vi "SUB_Get GUID.vi"() -> (0 "GUID OLE String":string, 1 "GUID String":string, 3 "GUID Cluster":T1 {"Data4" format="%.0x"; "Data3" format="%.0x"; "Data2" format="%.0x"; "Data1" format="%.0x"})   [LabVIEW 2015]
doc: "GUID stands for <B>G</B>lobally <B>U</B>nique <B>ID</B>entifier, a 128-bit integer used as unique identifier.\n\nThis VI makes a call to ole32.dll to create an absolutely unique number that you can use as a persistent identifier in a distributed environment.To a very high degree of certainty, this function returns a unique value: no other invocation, on the same or any other system (networked or not), should return the same value.\n\n<B>GUID Cluster</B> returns the GUID in a cluster that follows the GUID format.\n\n<B>GUID String</B> has the GUID as a string of characters.\n\n<B>GUID OLE String</B> has a format like that of the following sample:\n\n{c200e360-38c5-11ce-ae62-08002b2b79ef} \n \nwhere the successive fields break the GUID into the form:\n\nDWORD-WORD-WORD-WORD-WORD-DWORD\n\ncovering the 128-bit GUID. The string includes the enclosing braces, which are an OLE convention.\n\nEnrique Vargas\nvargas@jyestudio.com"
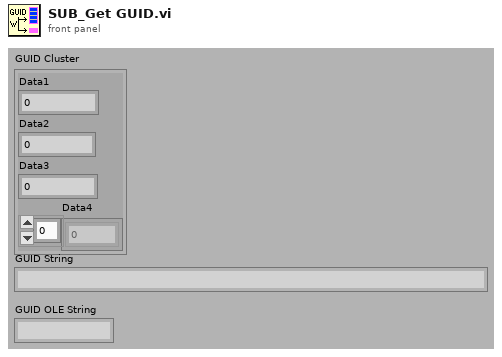
[diagram p1: front panel]
types:
  T1 = cluster{"Data1":u32, "Data2":u16, "Data3":u16, "Data4":u8[]}
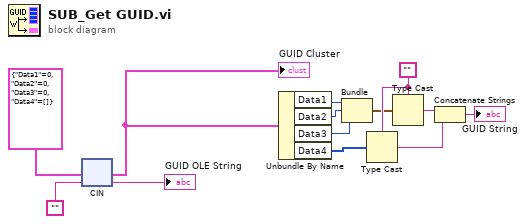
[diagram p0: block diagram]
diagram:
  w6 = ""
  n1 = cin(T1 {"Data1"=0, "Data2"=0, "Data3"=0, "Data4"=[]} ("GUID"), "") -> (w2:T1, →"GUID OLE String":string)
  "GUID Cluster" <- w2
  n2 = Unbundle By Name(w2) -> ("Data1"=w10:u32, "Data2"=w9:u16, "Data3"=w8:u16, "Data4"=w4:u8[])
  n3 = Bundle("Data1"=w10, "Data2"=w9, "Data3"=w8) -> (w3:cluster{"Data1":u32, "Data2":u16, "Data3":u16})  [unwired: 1 in]
  n4 = Type Cast(type=w6, x=w4) -> (*(type *) &x=w5:string)
  n5 = Type Cast(type=w6, x=w3) -> (*(type *) &x=w7:string)
  n6 = Concatenate Strings(w7, w5) -> (→"GUID String":string)
